vi "Process.vi"(0 "reference in":refnum<class "Simulated-PowerModule.lvclass">, 5 "error in":errorcluster) -> (14 "reference out":refnum<class "Simulated-PowerModule.lvclass">, 19 "error out":errorcluster)   [LabVIEW 2023, in "Simulated-PowerModule.lvlib" / "Simulated-PowerModule.lvclass"]
uses:
  Simulated-PowerModule.lvclass
  builds/PowerModuleInterface/PowerModuleInterface.lvlibp/Classes/PowerModule_interface/Slew Rates.ctl
  <instrlib>/HPS-17000/Client Facing Datatypes/Multi-Cycler Events.ctl
  <instrlib>/HPS-17000/Client Facing Datatypes/Heartbeat Event Data.ctl
  <instrlib>/HPS-17000/Client Facing Datatypes/Faults Event Data.ctl
  <instrlib>/HPS-17000/Client Facing Datatypes/Network Sync Event Data.ctl
  <instrlib>/HPS-17000/Client Facing Datatypes/Setpoint Stream Status Data.ctl
  builds/PowerModuleInterface/PowerModuleInterface.lvlibp/Classes/PowerModule_interface/Measurements.ctl
  <vilib>/addons/_JKI Toolkits/State Machine/_JKI_lib_State_Machine.llb/Conditional State String__jki_lib_state_machine.vi
  <vilib>/addons/_JKI Toolkits/State Machine/_JKI_lib_State_Machine.llb/Periodic Trigger__ogtk__JKI-SM__jki_lib_state_machine.vi
  Simulated-PowerModule.lvclass/Simulated-PowerModule.ctl
  <vilib>/Utility/SystemLogging/NI_SystemLogging.lvlib
  <instrlib>/HPS-17000/HPS-17000.lvclass
  builds/PowerModuleInterface/PowerModuleInterface.lvlibp/Classes/PowerModule_interface/PowerModuleInterface.lvclass
  <vilib>/measure/NI_MABase.lvlib
panel:
  in  "Main Tab Control":enum32{"CONFIG", "DEBUG"}(tab)
  out "Slew Rates":T1
  out "Last Command":string
  out "error info":errorcluster
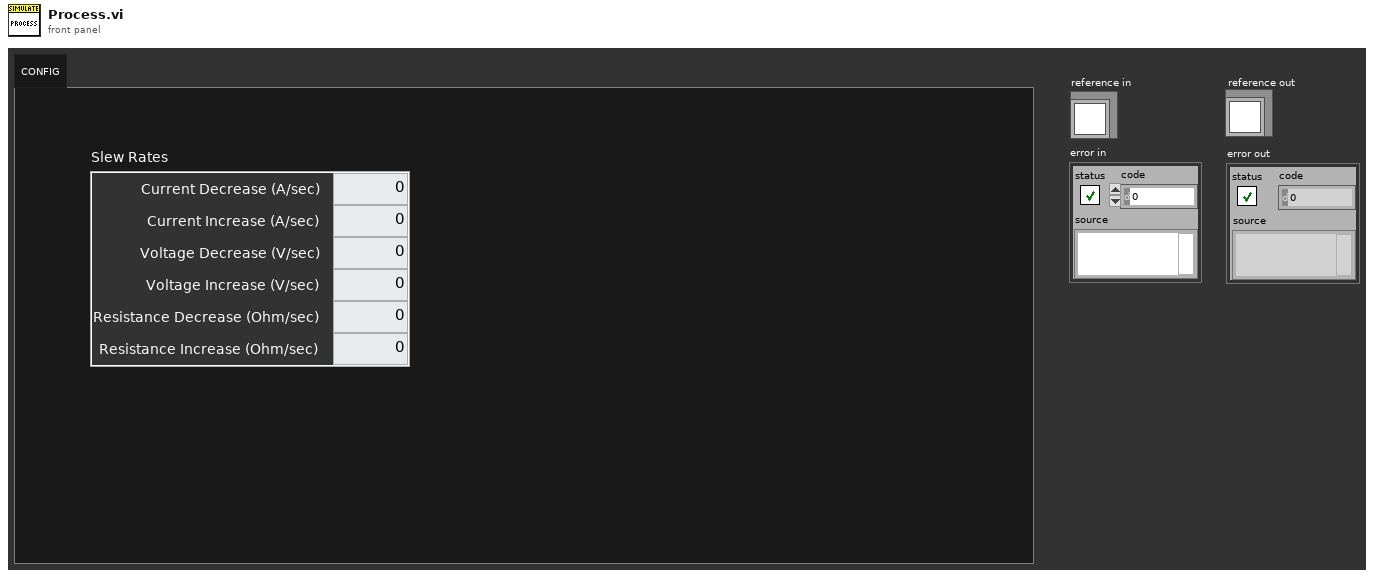
[diagram p1: front panel]
types:
  T1 = typedef "PowerModuleInterface.lvlibp/PowerModuleInterface.lvclass/Slew Rates.ctl" = cluster{"Current Decrease (A/sec)":dbl, "Current Increase (A/sec)":dbl, "Voltage Decrease (V/sec)":dbl, "Voltage Increase (V/sec)":dbl, "Resistance Decrease (Ohm/sec)":dbl, "Resistance Increase (Ohm/sec)":dbl}
  T2 = cluster{"Core":cluster{"Timeout":i32, "Events":cluster{"EventsToProcess":refnum<event-registration>, "UserEvents":refnum<event-registration>}, "EventFromProcess":refnum<user-event>, "ProcessSyncQueue":refnum<queue>, "QueueFromProcess":refnum<queue>, "Command":string, "Data":variant}}
  T3 = typedef "PowerModuleInterface.lvlibp/PowerModuleInterface.lvclass/Measurements.ctl" = cluster{"measured voltage (V)":dbl, "measured current (A)":dbl, "setpoint voltage (V)":dbl, "setpoint current (A)":dbl, "timestamp":dbl}
  T4 = enum32{"Invalid", "Standard", "Closed", "Hidden", "Minimized", "Maximized"}
  T5 = cluster{"EventsToProcess":refnum<event-registration>, "UserEvents":refnum<event-registration>}
  T6 = typedef "Simulated-PowerModule.lvlib/Simulated-PowerModule.lvclass/ObjectAttributes.ctl" = cluster{"JSON Config Path":path, "mode":T7, "Configuration":T8, "connected":bool, "reserved":bool, "energized":bool, "output enabled":bool, "setpoint":cluster{"voltage":dbl, "current":dbl, "resistance":dbl}, "last timestamp":i64, "measurement array":T3[], "profile":dbl[][], "step dt":i64, "measurement array size":u32}
  T7 = typedef "Simulated-PowerModule.lvlib/Simulated-PowerModule.lvclass/Mode.ctl" = u16
  T8 = typedef "Simulated-PowerModule.lvlib/Simulated-PowerModule.lvclass/Configuration.ctl" = cluster{"range":T9, "Limits":T10}
  T9 = typedef "PowerModuleInterface.lvlibp/PowerModuleInterface.lvclass/Range.ctl" = cluster{"Current Max (A)":dbl, "Current Min (A)":dbl, "Voltage Max (V)":dbl, "Voltage Min (V)":dbl}
  T10 = typedef "PowerModuleInterface.lvlibp/PowerModuleInterface.lvclass/Limits.ctl" = cluster{"Current Max (A)":dbl, "Current Min (A)":dbl, "Voltage Max (V)":dbl, "Voltage Min (V)":dbl, "Power Max (W)":dbl, "Power Min (W)":dbl}
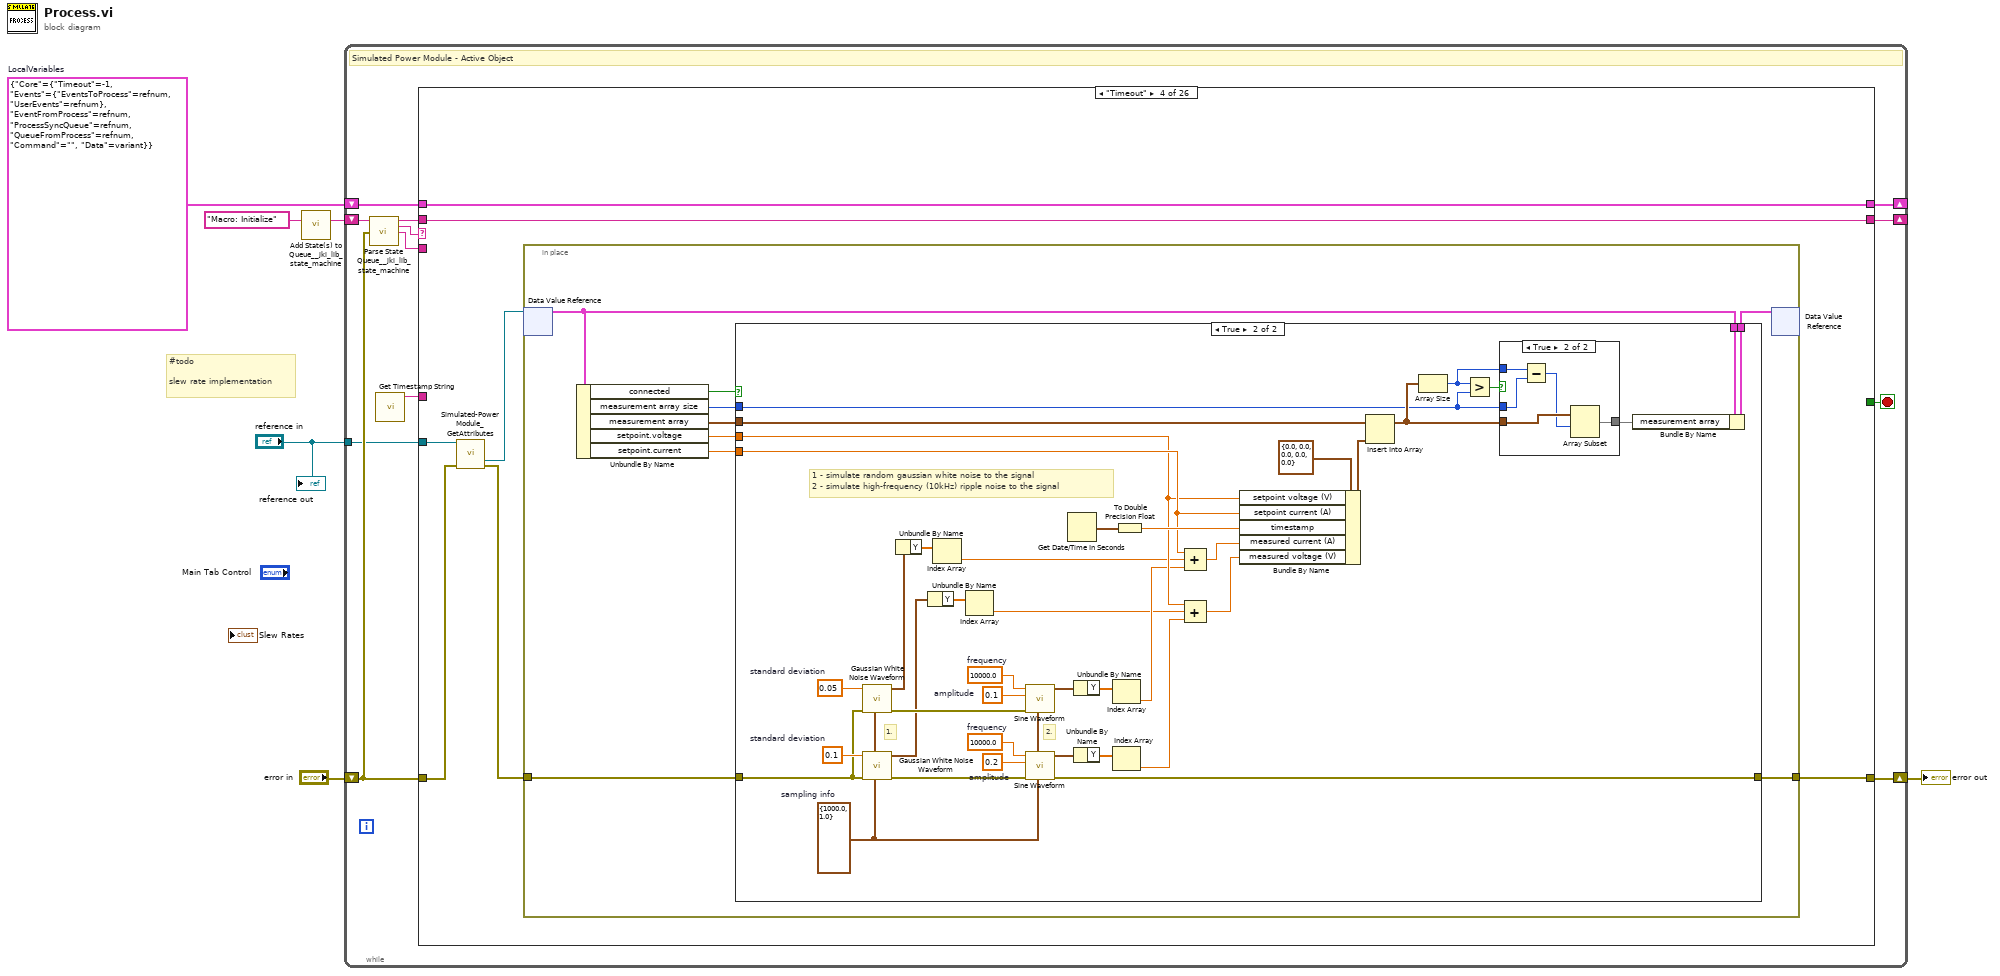
[diagram p0: block diagram]
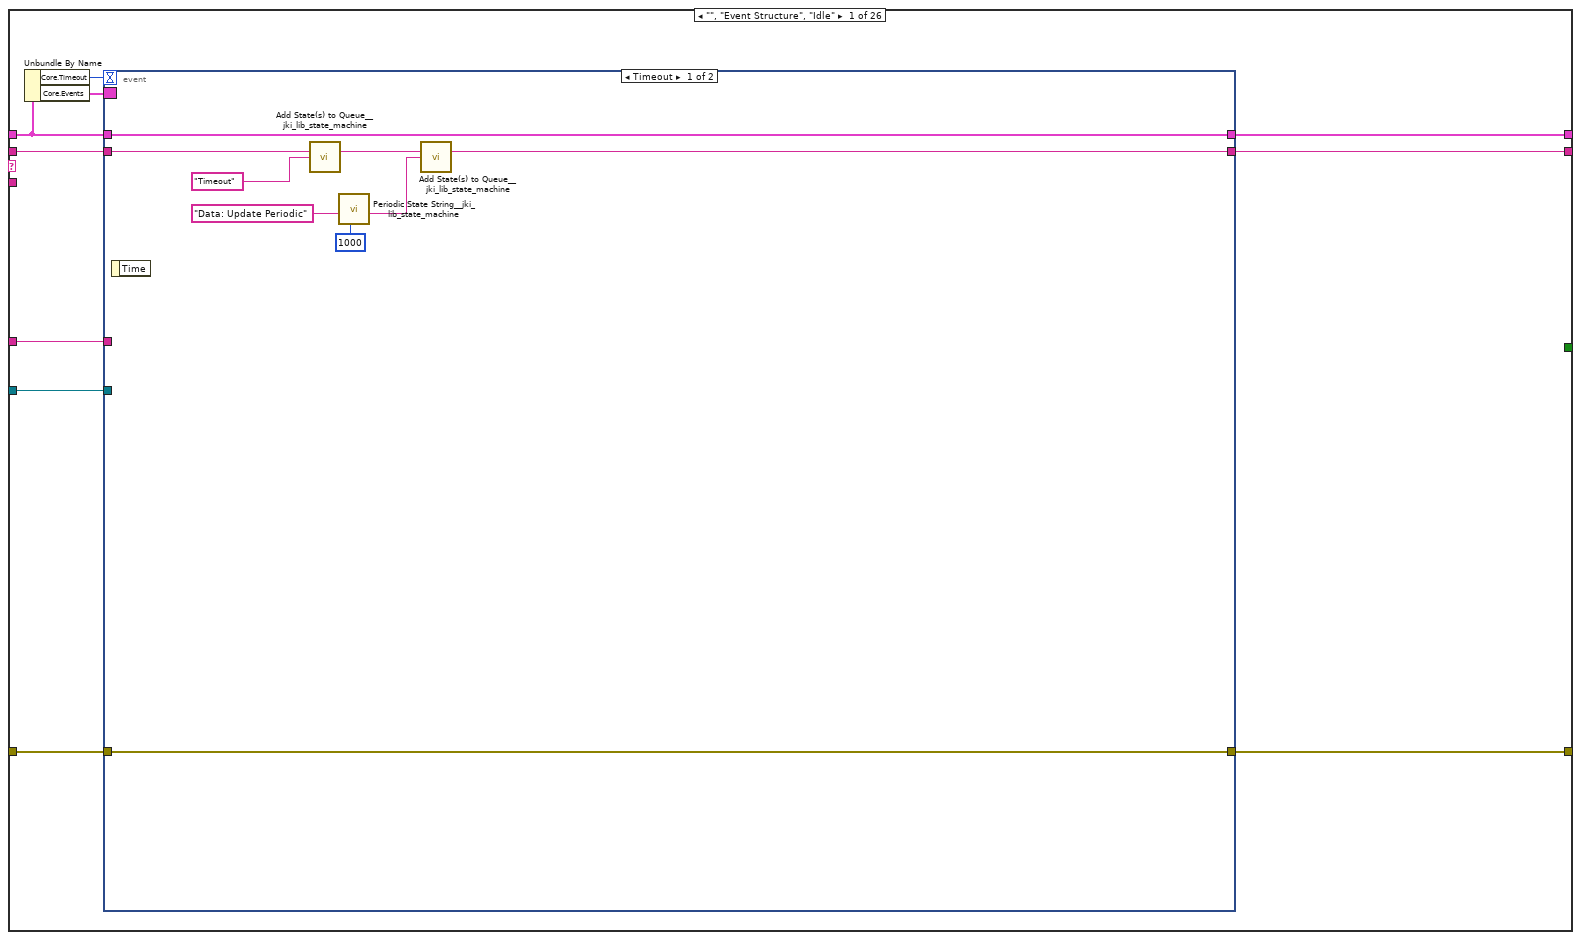
[diagram p2: hidden frame]
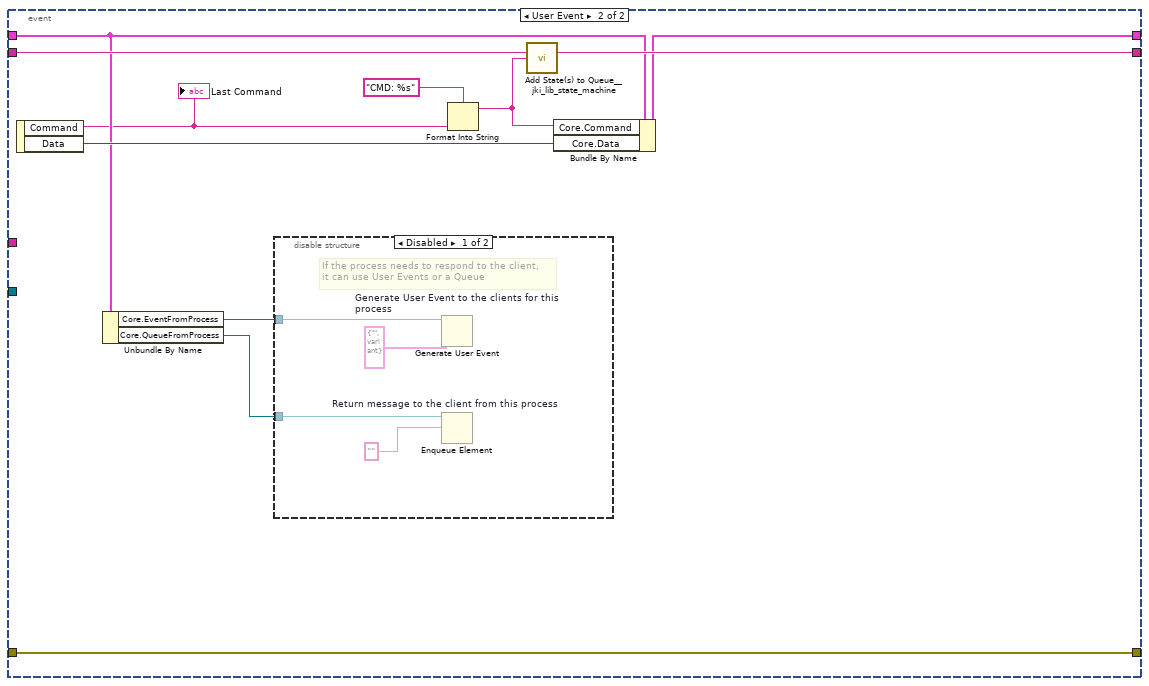
[diagram p3: hidden frame]
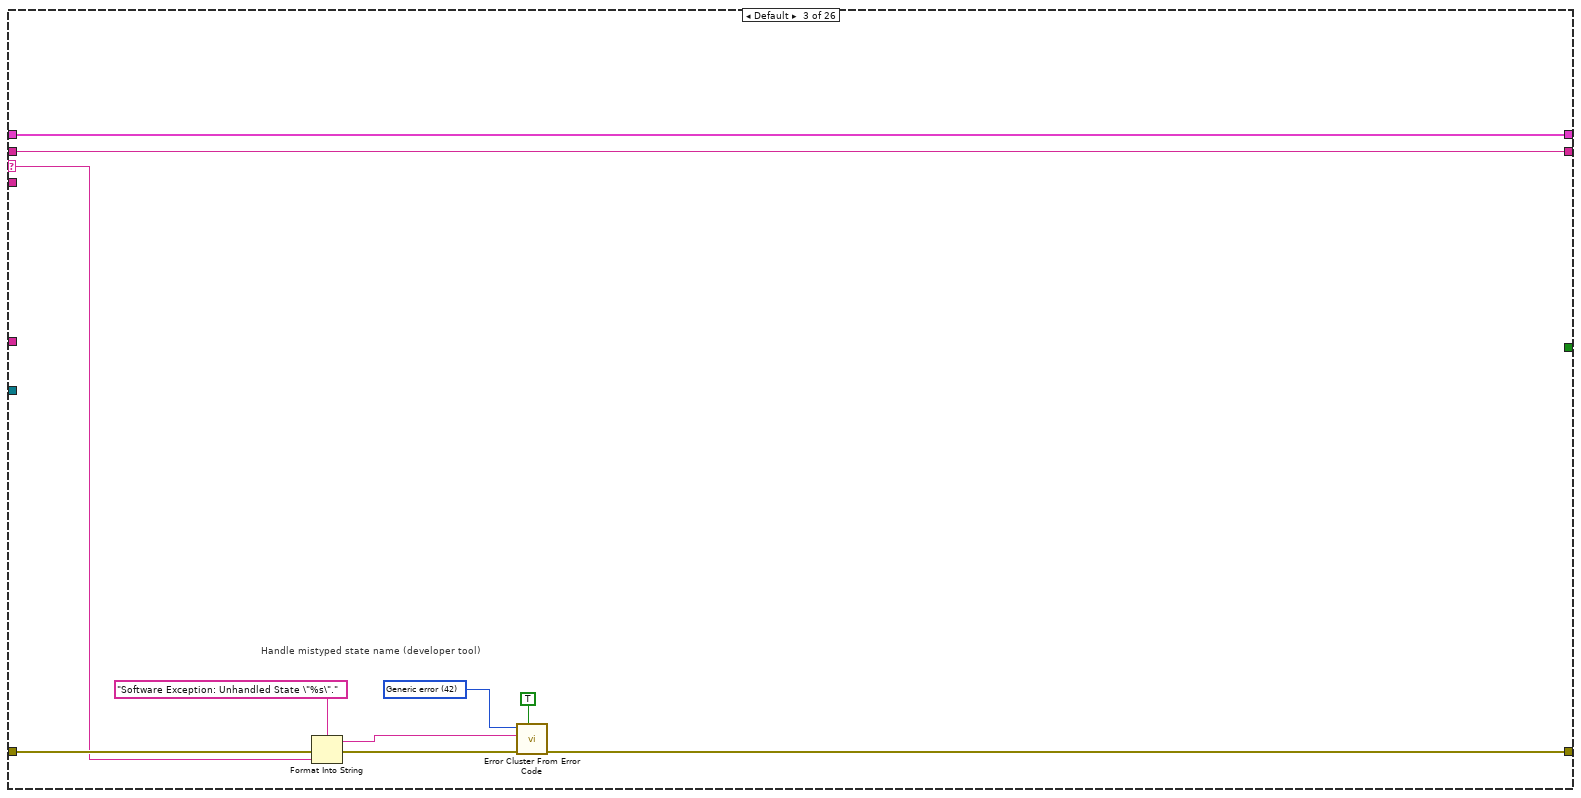
[diagram p6: hidden frame]
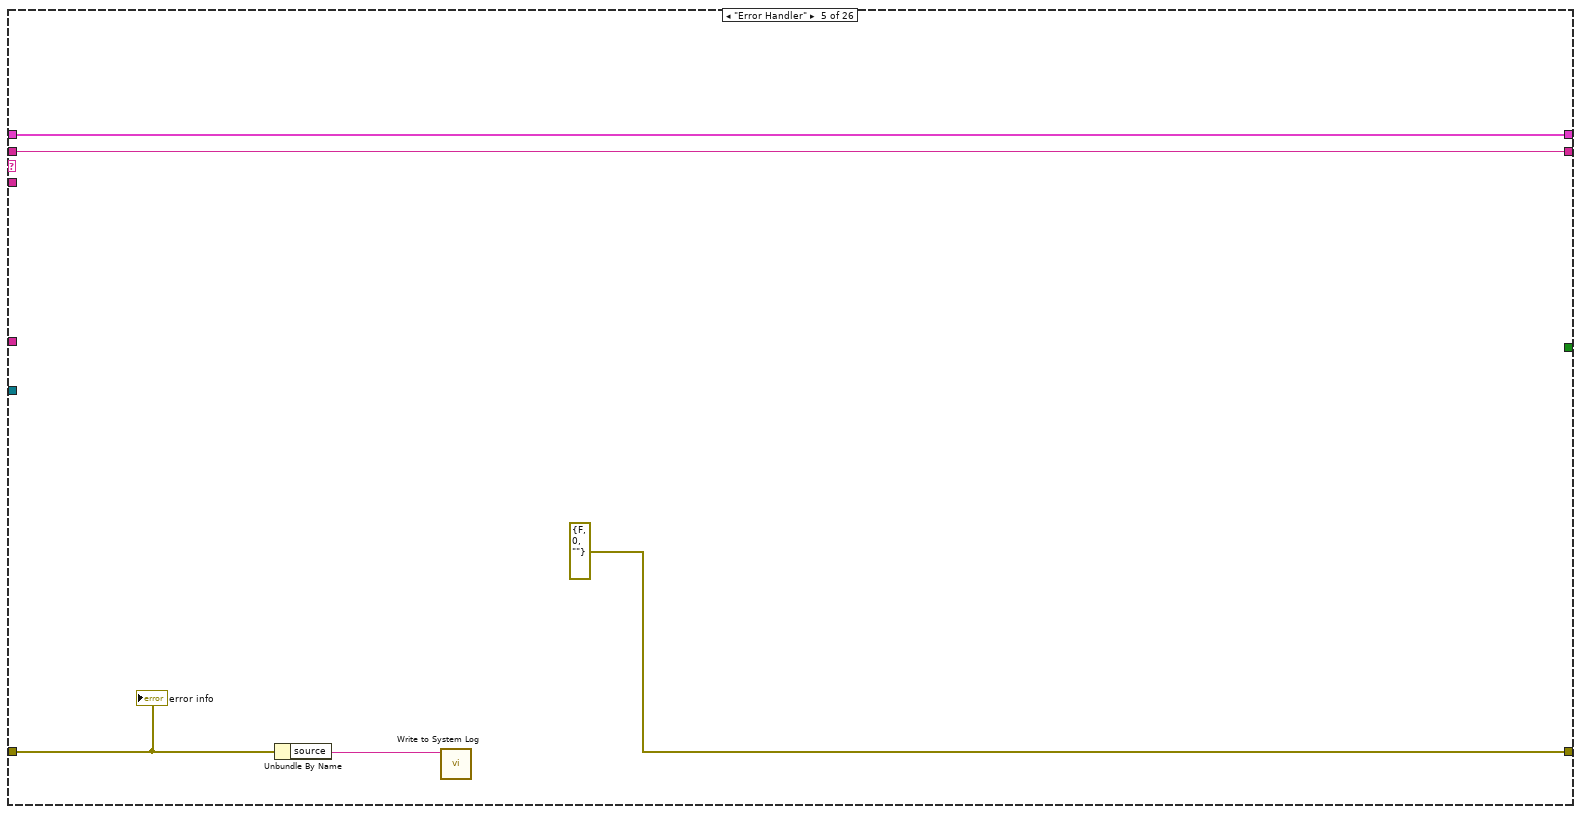
[diagram p9: hidden frame]
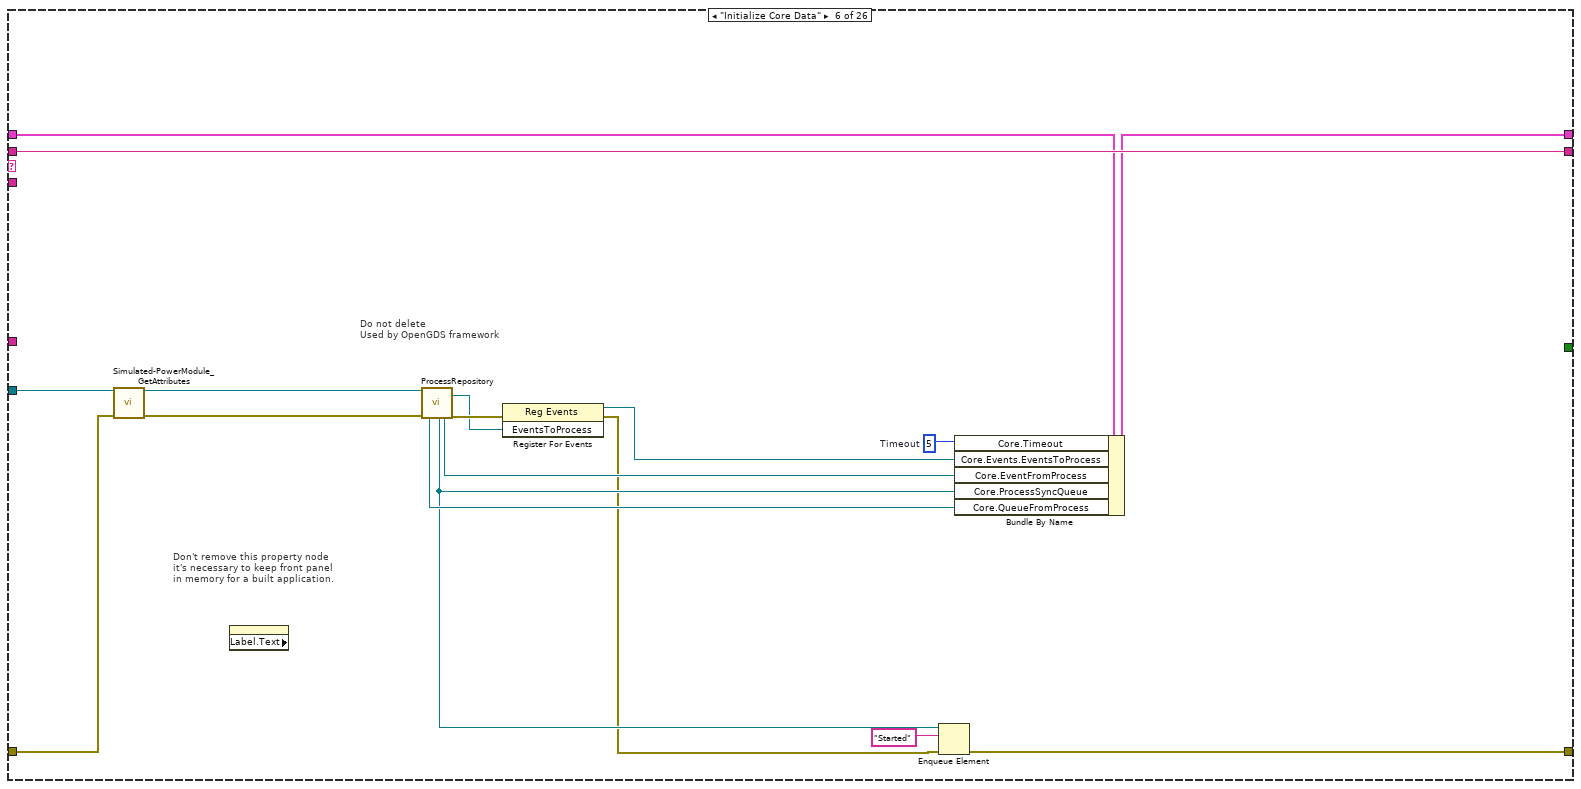
[diagram p10: hidden frame]
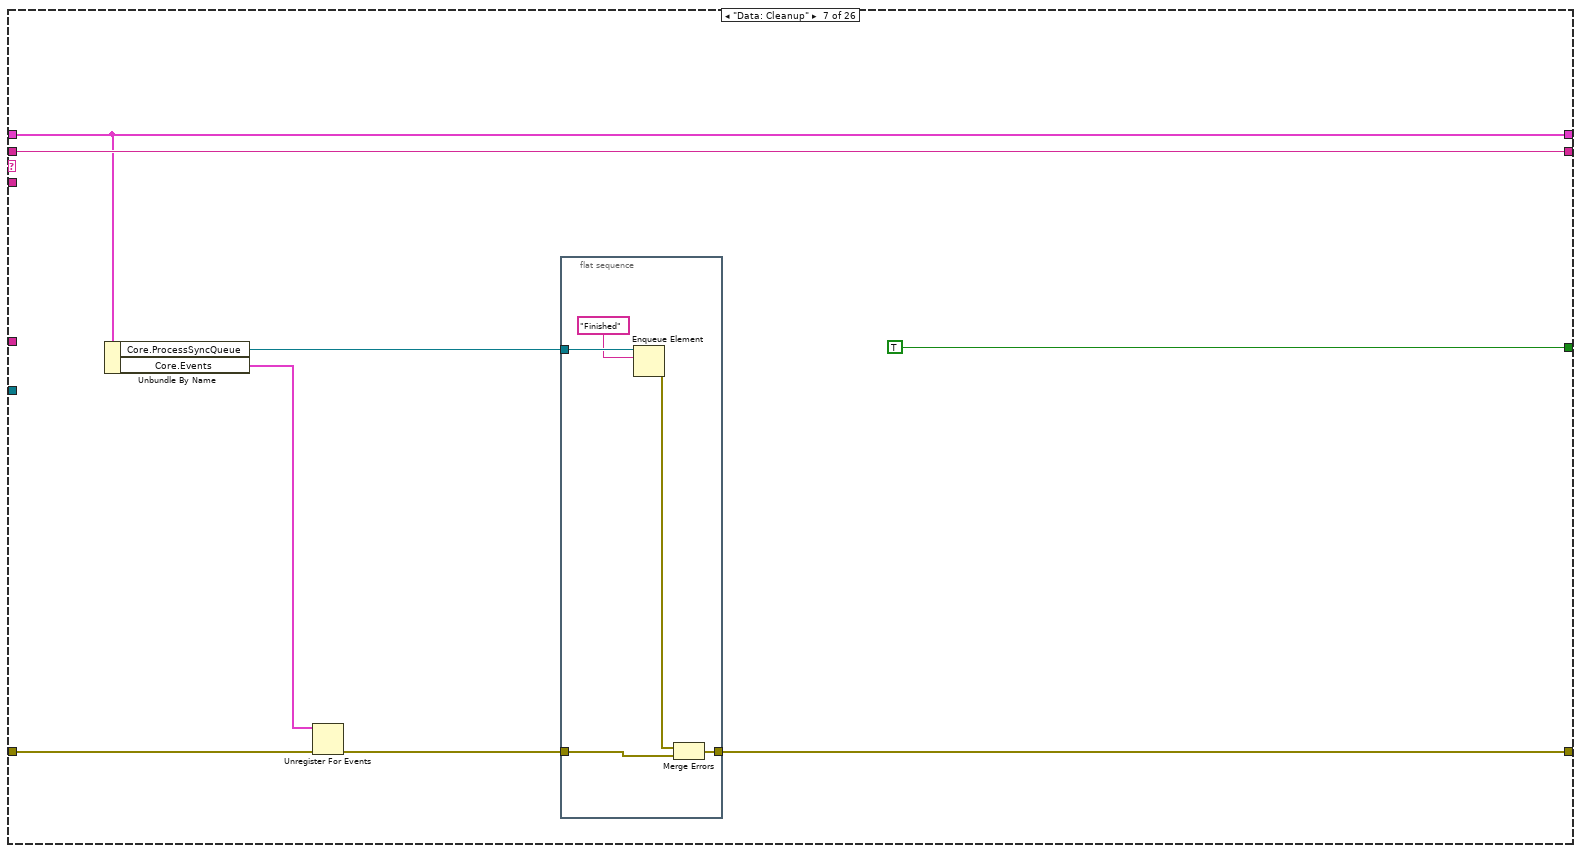
[diagram p11: hidden frame]
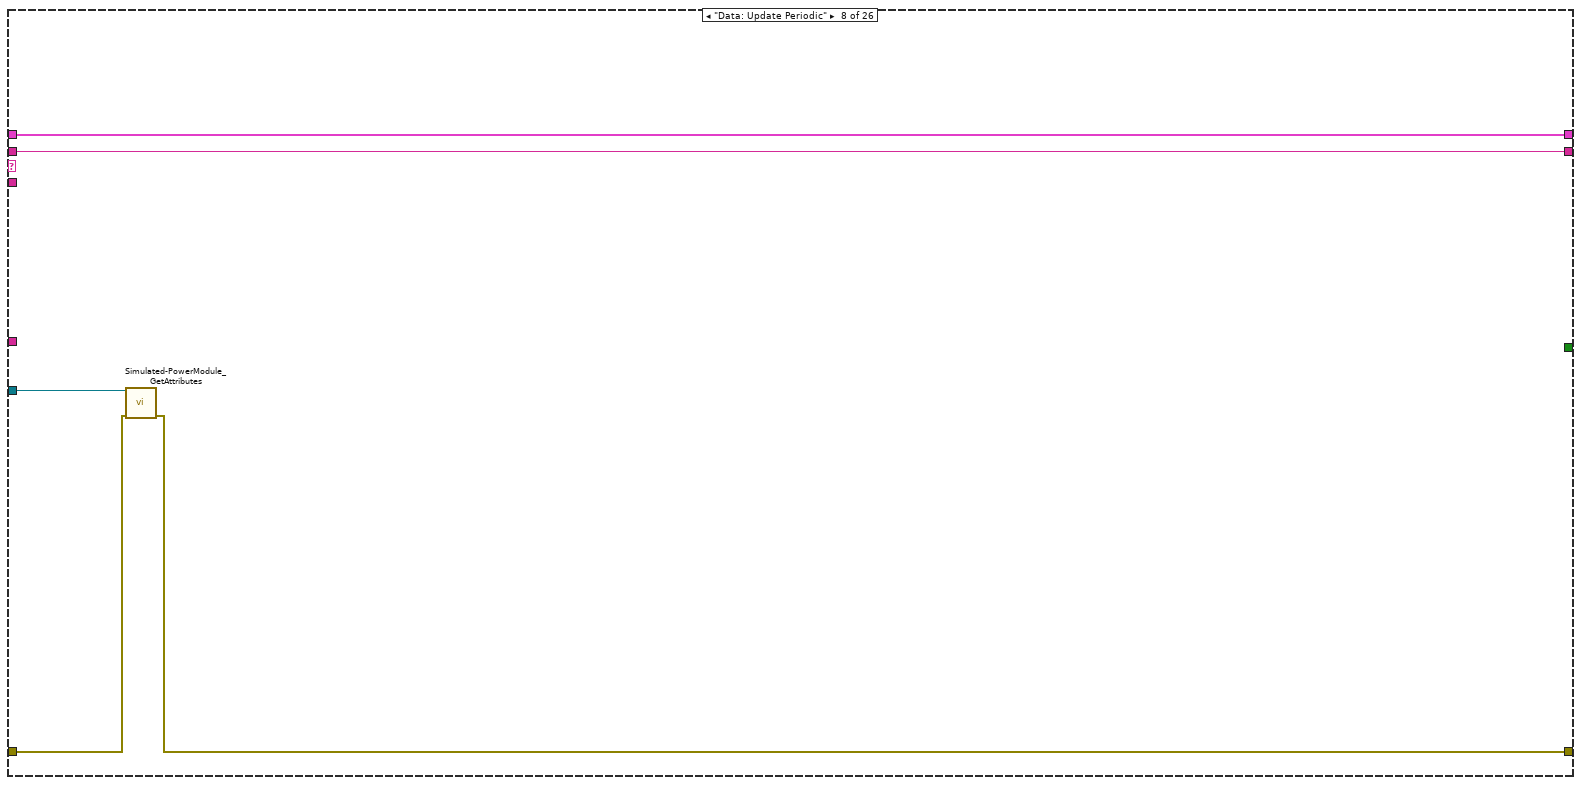
[diagram p12: hidden frame]
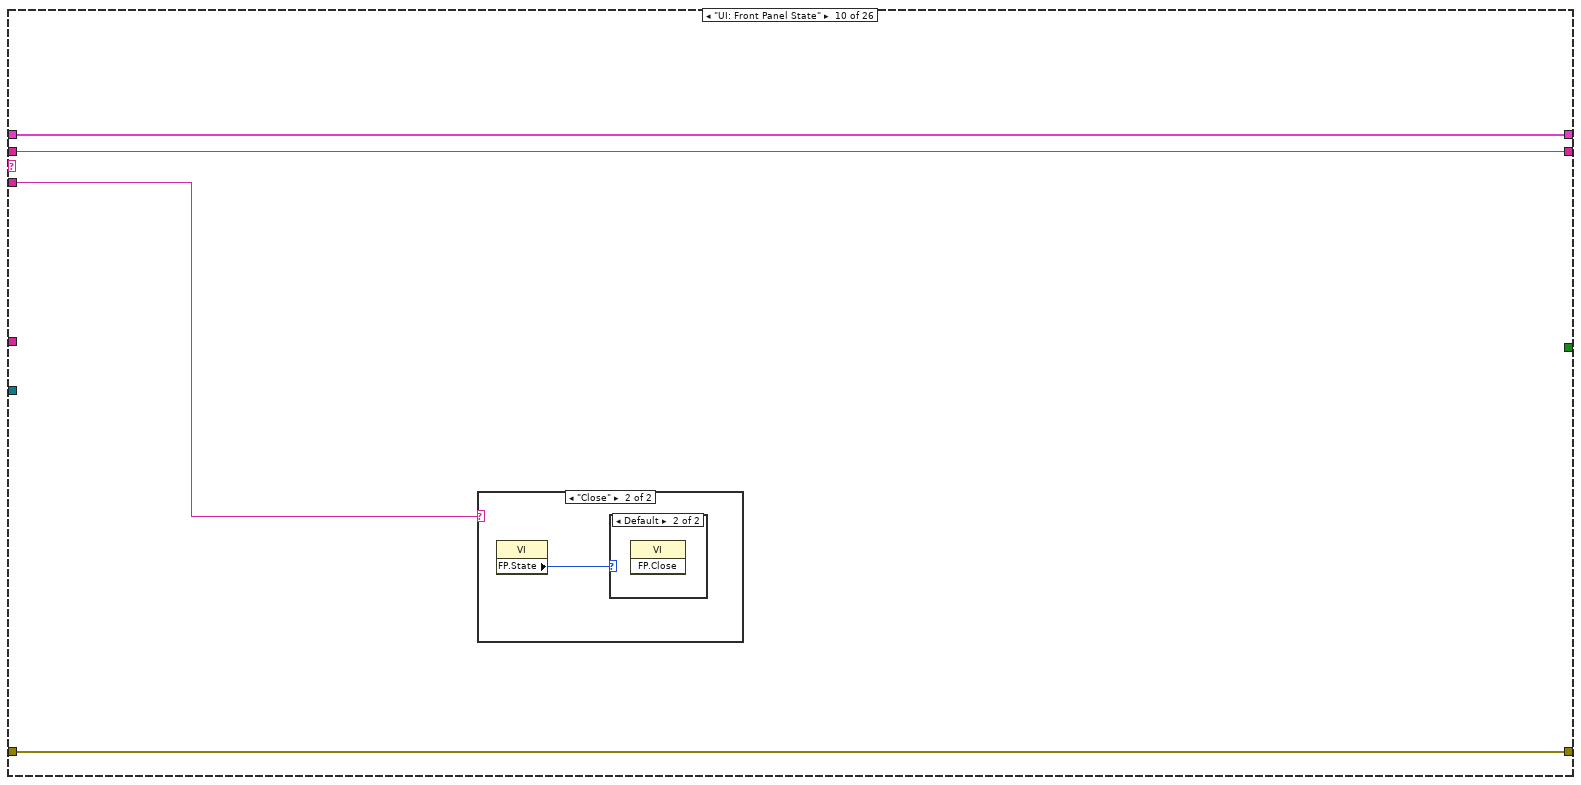
[diagram p14: hidden frame]
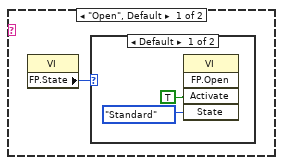
[diagram p15: hidden frame]
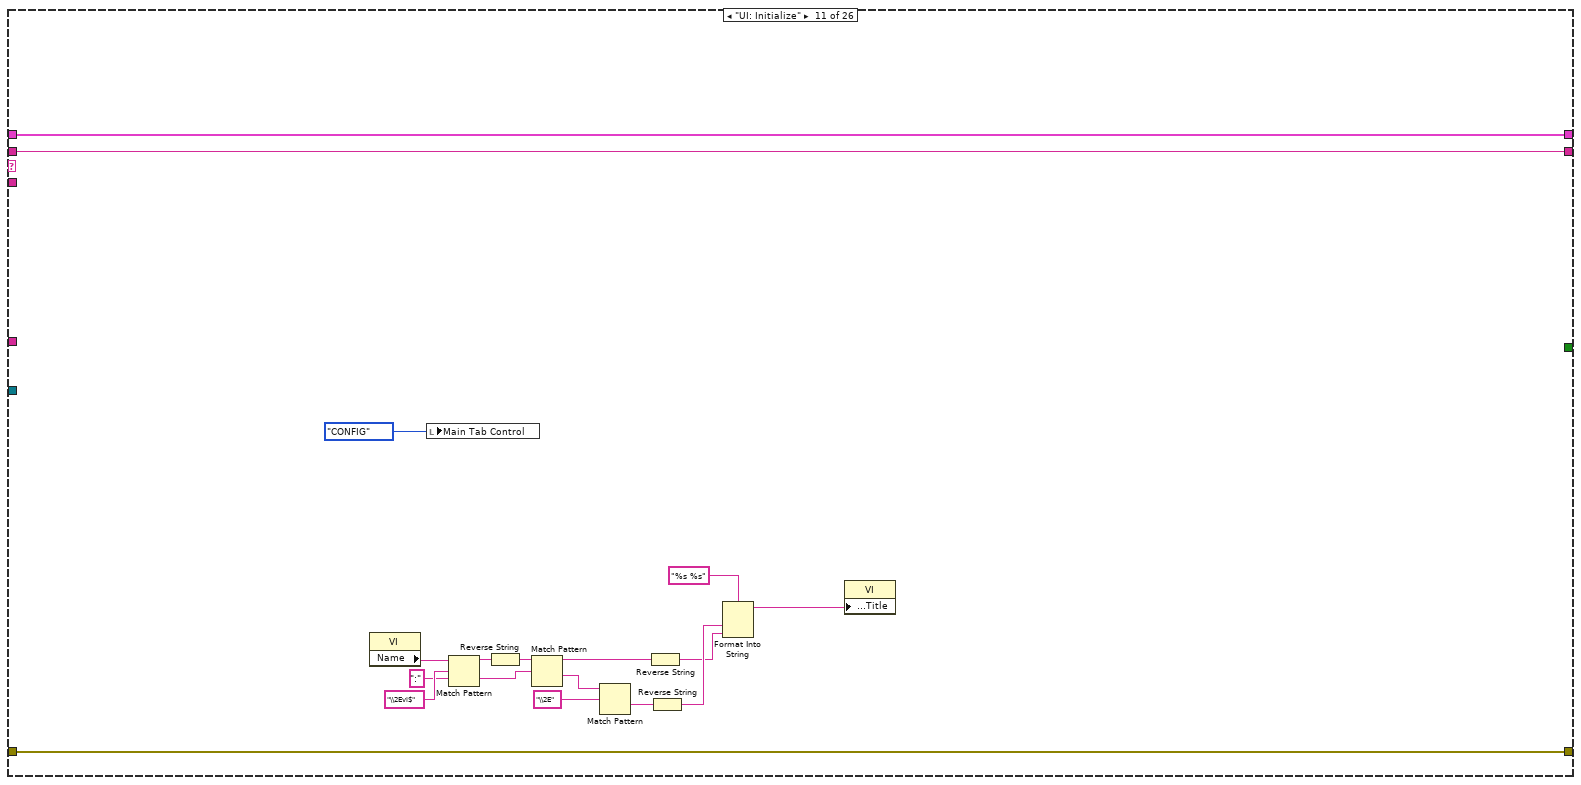
[diagram p18: hidden frame]
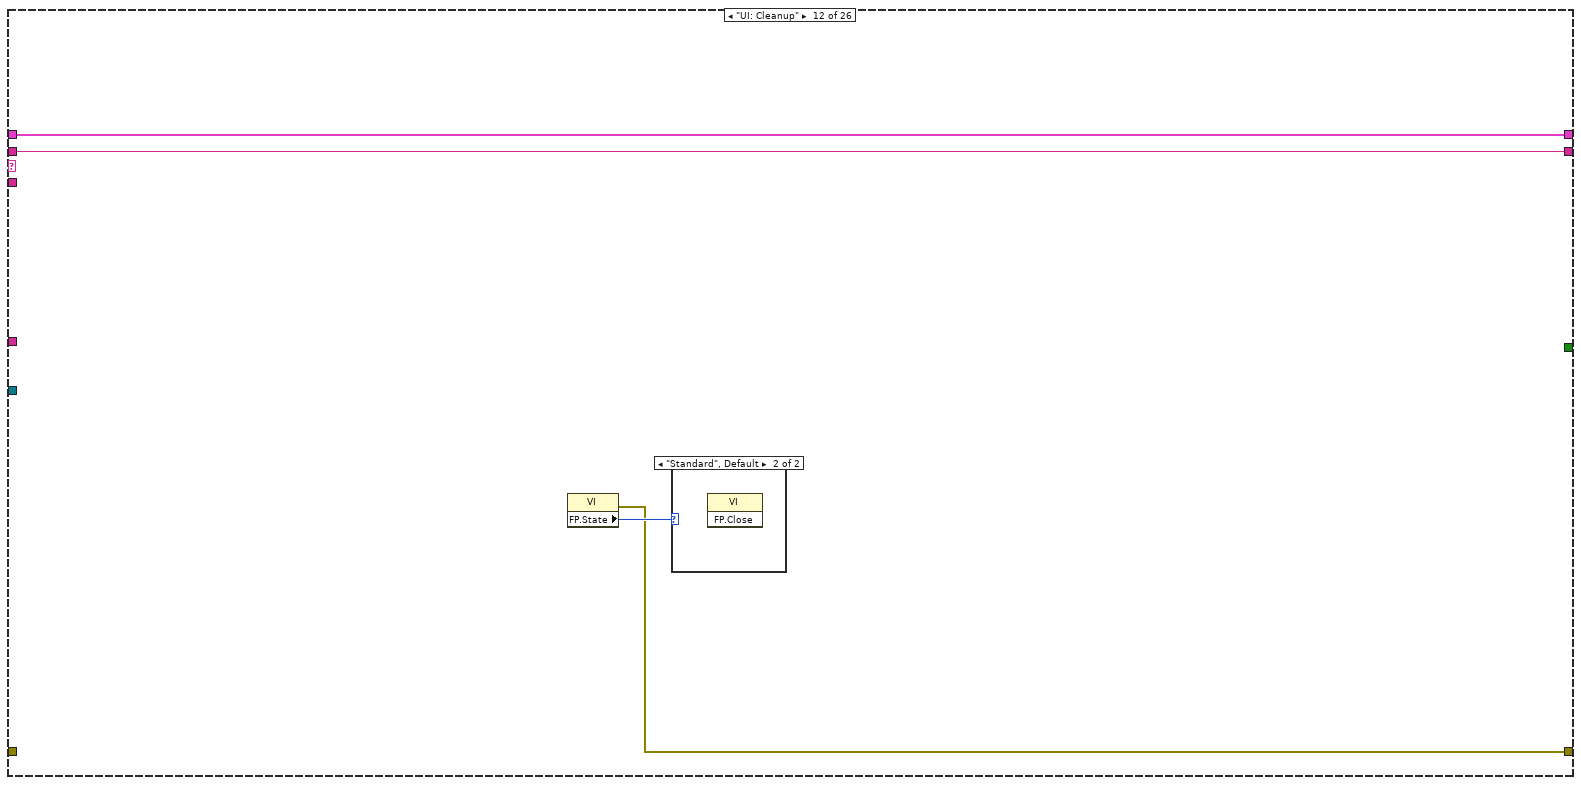
[diagram p19: hidden frame]
diagram:
  w6 = T2 {"Core"={"Timeout"=-1, "Events"={"EventsToProcess"=refnum, "UserEvents"=refnum}, "EventFromProcess"=refnum, "ProcessSyncQueue"=refnum, "QueueFromProcess"=refnum, "Command"="", "Data"=variant}}  # LocalVariables
  # "#todo\n\nslew rate implementation"
  n1 = call <vilib>:"Add State(s) to Queue__jki_lib_state_machine.vi"("State(s) in (\"\")"="Macro: Initialize" ("States Out")) -> ("States Out"=w2:string)  [unwired: 14 in]
  n2 = while {
    shift-right: [w17] -> w5
    shift-left: "error in" -> [w18]
    shift-right: [w10] -> _
    shift-left: w2 -> [w13]
    shift-right: [w16] -> _
    shift-left: w6 -> [w15]
    tunnel: "reference in" -> [w8]
    stop <- w9 stop-if-true
    # "Simulated Power Module - Active Object"
    n3 = call <vilib>:"Parse State Queue__jki_lib_state_machine.vi"("State Queue"=w13, "Error In (no error)"=w18) -> ("Remaining States"=w12:string, "Current State"=w14:string, "Arguments"=w11:string)  [unwired: 11 in]
    n4 = call "Get Timestamp String.vi"() -> ("date/time string"=w7:string)  [unwired: 11 in]
    n5 = case shown="\"Timeout\"" w14 {
      selector: w14 -> [_ _ w56 _ _ _ _ _ _ _ _ _ _ _ _ _ _ _ _ _ _ _ _ _ _ _]
      tunnel: w18 -> [w24 w55 w58 w69 w131 w135 w152 w165 w171 w172 w196 _ w202 w216 w219 w222 w227 w232 w235 w242 w251 w253 w263 w266 w271 w276]
      tunnel: [w22 w55 w57 w66 errorcluster {"status"=FALSE, "code"=0, "source"=""} ("error constant") w150 w154 w164 w171 w172 w196 w197 w201 w216 w219 w222 w227 w232 w235 w242 w246 w257 w263 w266 w271 w276] -> w17
      tunnel: [w28 w54 w65 w71 w133 w148 w155 w167 w170 w174 w188 w198 w205 w215 w218 w221 w226 w231 w234 w241 w250 w259 w262 w265 w270 w275] -> w16
      tunnel: w15 -> [w25 w54 w65 w71 w133 w147 w155 w167 w170 w174 w188 w198 w205 w215 w218 w221 w226 w231 w234 w241 w250 w259 w262 w265 w270 w275]
      tunnel: w12 -> [w27 w53 w64 w72 w132 w149 w158 w168 w169 w175 w195 w200 w204 w214 w217 w220 w225 w230 _ w240 w252 w260 w261 w264 w269 w274]
      tunnel: w11 -> [_ _ _ _ _ _ _ _ _ w173 _ _ w203 _ _ _ _ _ _ w237 _ _ _ _ _ _]
      tunnel: [w26 w53 w64 w72 w132 w149 w158 w168 w169 w175 w195 w200 w204 w214 w217 w220 w224 w229 "Macro: Exit" ("State(s) at Back (\"\")") w239 w252 w260 w261 w264 w267 w273] -> w10
      tunnel: [_ _ _ _ _ _ TRUE _ _ _ _ _ _ _ _ _ _ _ _ _ _ _ _ _ _ _] -> w9
      tunnel: w8 -> [w19 _ _ w70 _ w138 _ w166 _ _ _ _ _ _ _ _ _ _ _ _ _ _ _ _ _ _]
      tunnel: w7 -> [w20 _ _ _ _ _ _ _ _ _ _ _ _ _ _ _ _ _ _ _ _ _ _ _ _ _]
      frame "", "Event Structure", "Idle" {
        n6 = Unbundle By Name(w25) -> ("Core.Timeout"=w23:i32, "Core.Events"=w21:T5)
        n7 = event shown="[0] Timeout" {
          selector: w21 -> [_ _]
          dyn-events: _ -> [_ _]
          timeout: w23 -> [_ _]
          tunnel: w25 -> [w37 w41]
          tunnel: [w37 w46] -> w28
          tunnel: [w29 w48] -> w26
          tunnel: w27 -> [w36 w47]
          tunnel: [w34 w42] -> w22
          tunnel: w24 -> [w34 w42]
          tunnel: w20 -> [_ _]
          tunnel: w19 -> [_ _]
          event Timeout {
            n8 = event-data() -> ()  [unwired: 1 in, 1 out]
            n9 = call <vilib>:"Add State(s) to Queue__jki_lib_state_machine.vi"("State(s) in (\"\")"=w36, "State(s) at Back (\"\")"="Timeout" ("State(s) at Back (\"\")")) -> ("States Out"=w32:string)  [unwired: 13 in]
            n10 = call <vilib>:"Periodic State String__jki_lib_state_machine.vi"("Period (ms)"=u32 1000, "State"="Data: Update Periodic") -> ("State Out"=w31:string)  [unwired: 9 in]
            n11 = call <vilib>:"Add State(s) to Queue__jki_lib_state_machine.vi"("State(s) in (\"\")"=w32, "State(s) at Back (\"\")"=w31) -> ("States Out"=w29:string)  [unwired: 13 in]
          }
          event User Event {
            n12 = event-data() -> ("Command"=w39:string, "Data"=w45:variant)  [unwired: 1 in]
            "Last Command" <- w39
            n13 = Unbundle By Name(w41) -> ("Core.EventFromProcess"=w44:refnum<user-event>, "Core.QueueFromProcess"=w43:refnum<queue>)
            n14 = disable-structure shown="Disabled" {
              disable-tunnel: w44 -> [w52 _]
              disable-tunnel: w43 -> [w51 _]
              frame Disabled {
                # "If the process needs to respond to the client,\nit can use User Events or a Queue"
                n15 = Generate User Event "Generate User Event to the clients for this process"(user event=w52, event data cluster=cluster{"Command":string, "Data":variant} {"Command"="", "Data"=variant} ("event data")) -> ()  [unwired: 2 in, 2 out]
                n16 = Enqueue Element "Return message to the client from this process"(queue=w51, element="") -> ()  [unwired: 2 in, 3 out]
              }
              frame Enabled {
              }
            }
            n17 = Format Into String(format string="CMD: %s", w39) -> (resulting string=w38:string)  [unwired: 2 in, 1 out]
            n18 = call <vilib>:"Add State(s) to Queue__jki_lib_state_machine.vi"("State(s) in (\"\")"=w47, "State(s) at Back (\"\")"=w38) -> ("States Out"=w48:string)  [unwired: 13 in]
            n19 = Bundle By Name(cluster=w41, "Core.Command"=w38, "Core.Data"=w45) -> (w46:T2)
          }
        }
      }
      frame "---------- Core ----------" {
      }
      frame Default {
        w62 = 42 items=["No error", "Argument error", "Memory is full", "Out of zone", "End of file", "File already open", "Generic file I/O error", "File not found", "File permission error", "Disk is full", "Duplicate path", "Too many files open", "System feature not enabled", "Resource file not found", "Cannot add resource", "Resource not found", "Image not found", "Image memory error", "Pen does not exist", "Config type invalid", "Config token not found", "Config parse error", "Config memory error", "Bad external code format", "Bad external code offset", "External code not present", "Null window", "Destroy window error", "Null menu", "Print aborted", "Bad print record", "Print driver error", "Windows error during printing", "Memory error during printing", "Print dialog error", "Generic print error", "Invalid device refnum", "Device not found", "Device parameter error", "Device unit error", "Cannot open device", "Device call aborted", "Generic error", "Cancelled by user", "Object ID too low", "Object ID too high", "Object not in heap", "Unknown heap", "Unknown object (invalid DefProc)", "Unknown object (DefProc not in table)", "Message out of range", "Invalid (null) method", "Unknown message", "Manager call not supported", "Bad address", "Network operation in progress", "Network operation timed out", "Connection is busy", "Network attribute not supported", "Network error", "Address in use", "System out of memory", "Connection aborted", "Connection refused", "Not connected", "Already connected", "Connection closed", "Initialization error (interapplication manager)", "Bad occurrence", "Wait on unbound occurrence handler", "Occurrence queue overflow", "Datalog type conflict", "Unused", "Unrecognized type (interapplication manager)", "Memory corrupt", "Failed to make temporary DLL", "Old CIN version", "Drag socket not found", "Failed to load drop-object", "Failed to register OLE object", "Failed to release OLE object", "Format specifier type mismatch", "Unknown format specifier", "Too few format specifiers", "Too many format specifiers", "Scan failed", "Newer CIN version", "Error converting to variant", "Runtime menu error", "Password tampered", "Variant attribute not found", "Incompatible variant data type", "Event data is not available", "Event Store is not present", "Occurrence is not found", "Event Queue is not created", "Event info is not available", "Refnum passed is NULL", "Error retrieving Class GUID", "Error retrieving CoClass GUID", "Error retrieving TypeLib GUID.", "Bad built application magic bytes.", "Specific driver is different from the specific driver associated with the Logical Name.", "There is no session opened to the class driver.", "Max Error", "MAX - Error with config objects", "MAX - Error loading configuration", "MAX - Group not supported"]
        # "Handle mistyped state name (developer tool)"
        n20 = Format Into String(format string="Software Exception: Unhandled State \"%s\"." ("message"), error in=w58, w56) -> (resulting string=w61:string, error out=w60:errorcluster)  [unwired: 1 in]
        n21 = call <vilib>:"Error Cluster From Error Code.vi"("show call chain? (False)"=TRUE, "error in (no error)"=w60, "error message (\"\")"=w61, "error code (0)"=w62) -> ("error out"=w57:errorcluster)  [unwired: 5 in]
      }
      frame "Timeout" {
        # "High-Speed Measurement Stream"
        n22 = call "Simulated-PowerModule_GetAttributes.vi"("reference in"=w70, "Error In"=w69) -> ("DataRef"=w68:refnum<data-value>, "Error Out"=w67:errorcluster)  [unwired: 10 in, 2 out]
        n23 = in-place {
          in-place-border: w67 -> [w74]
          in-place-border: [w73] -> w66
          n24 = in-place-dvr #1(w68) -> (w80:T6)  [unwired: 1 out]
          n25 = Unbundle By Name(w80) -> ("connected"=w75:bool, "measurement array size"=w78:u32, "measurement array"=w79:T3[], "setpoint.voltage"=w76:dbl, "setpoint.current"=w77:dbl)
          n26 = case shown="True" w75 {
            tunnel: [w83 w122] -> w81
            tunnel: w80 -> [w83 w121]
            tunnel: w79 -> [_ w120]
            tunnel: w78 -> [_ w113]
            tunnel: w77 -> [_ w108]
            tunnel: w76 -> [_ w103]
            tunnel: w74 -> [w82 w96]
            tunnel: [w82 w106] -> w73
            frame False {
            }
            frame True {
              w95 = 0.05  # standard deviation
              w98 = 10000.0  # frequency
              w97 = 0.1  # amplitude
              w104 = 10000.0  # frequency
              w105 = 0.2  # amplitude
              w110 = 0.1  # standard deviation
              w93 = cluster{"Fs":dbl, "#s":dbl} {"Fs"=1000.0, "#s"=1.0}  # sampling info
              # "1 - simulate random gaussian white noise to the signal\n2 - simulate high-frequency (10kHz) ripple noise to the signal"
              # "2."
              # "1."
              n27 = call <vilib>:"Gaussian White Noise Waveform.vi"("sampling info"=w93, "error in (no error)"=w96, "standard deviation"=w95) -> ("error out"=w94:errorcluster, "signal out"=w89:waveform(dbl))  [unwired: 7 in]
              n28 = call <vilib>:"Gaussian White Noise Waveform.vi"("sampling info"=w93, "error in (no error)"=w96, "standard deviation"=w110) -> ("error out"=w107:errorcluster, "signal out"=w87:waveform(dbl))  [unwired: 7 in]
              n29 = Unbundle By Name(w89) -> ("Y"=w109:dbl[])
              n30 = Unbundle By Name(w87) -> ("Y"=w86:dbl[])
              n31 = Index Array(array=w109) -> (element=w92:dbl)  [unwired: 1 in]
              n32 = Index Array(array=w86) -> (element=w85:dbl)  [unwired: 1 in]
              n33 = call <vilib>:"Sine Waveform.vi"("sampling info"=w93, "error in (no error)"=w94, "amplitude"=w97, "frequency"=w98) -> ("signal out"=w90:waveform(dbl))  [unwired: 6 in, 1 out]
              n34 = call <vilib>:"Sine Waveform.vi"("sampling info"=w93, "error in (no error)"=w107, "amplitude"=w105, "frequency"=w104) -> ("error out"=w106:errorcluster, "signal out"=w100:waveform(dbl))  [unwired: 6 in]
              n35 = Get Date/Time In Seconds() -> (seconds since 1Jan1904=w112:timestamp)
              n36 = Unbundle By Name(w90) -> ("Y"=w91:dbl[])
              n37 = Unbundle By Name(w100) -> ("Y"=w99:dbl[])
              n38 = Index Array(array=w91) -> (element=w88:dbl)  [unwired: 1 in]
              n39 = Index Array(array=w99) -> (element=w84:dbl)  [unwired: 1 in]
              n40 = To Double Precision Float(number=w112) -> (double precision float=w111:dbl)
              n41 = Compound Arithmetic op=ADD(w108, w92, w88) -> (w102:dbl)
              n42 = Compound Arithmetic op=ADD(w103, w85, w84) -> (w101:dbl)
              n43 = Bundle By Name(cluster=T3 {"measured voltage (V)"=0.0, "measured current (A)"=0.0, "setpoint voltage (V)"=0.0, "setpoint current (A)"=0.0, "timestamp"=0.0} ("Measurements"), "setpoint voltage (V)"=w103, "setpoint current (A)"=w108, "timestamp"=w111, "measured current (A)"=w102, "measured voltage (V)"=w101) -> (w115:T3)
              n44 = Insert Into Array(array=w120, new element=w115) -> (w117:T3[])  [unwired: 1 in]
              n45 = Array Size(array=w117) -> (size(s)=w114:i32)
              n46 = Greater?(x=w114, y=w113) -> (0:w116:bool)
              n47 = case shown="True" w116 {
                tunnel: [w123 w128] -> w119
                tunnel: w117 -> [w123 w127]
                tunnel: w114 -> [_ w126]
                tunnel: w113 -> [_ w125]
                frame False {
                }
                frame True {
                  n48 = Subtract(x=w126, y=w125) -> (x-y=w124:u32)
                  n49 = Array Subset(array=w127, index=w124) -> (w128:T3[])  [unwired: 1 in]
                }
              }
              n50 = Bundle By Name(cluster=w121, "measurement array"=w119) -> (w122:T6)
            }
          }
          n51 = in-place-dvr #1(w81) -> ()  [unwired: 2 out]
        }
      }
      frame "Error Handler" {
        n52 = Unbundle By Name(w131) -> ("source"=w129:string)
        n53 = call <vilib>:"Write to System Log.vi"("message"=w129) -> ()  [unwired: 10 in, 1 out]
        "error info" <- w131
      }
      frame "Initialize Core Data" {
        w139 = 5  # Timeout
        # "Do not delete\nUsed by OpenGDS framework"
        # "Don't remove this property node\nit's necessary to keep front panel\nin memory for a built application."
        # "Template created by VI Technologies"
        n54 = call "Simulated-PowerModule_GetAttributes.vi"("reference in"=w138, "Error In"=w135) -> ("reference out"=w136:refnum<class "Simulated-PowerModule.lvclass">, "Error Out"=w137:errorcluster)  [unwired: 10 in, 2 out]
        n55 = property on="reference in" class="LVClassControl (strict)" props=["Label", "Text"]() -> ()  [unwired: 2 in, 3 out]
        n56 = call "ProcessRepository.vi"("reference in"=w136, "Error In"=w137) -> ("QueueFromProcess"=w142:refnum<queue>, "ProcessSyncQueue"=w140:refnum<queue>, "EventFromProcess"=w143:refnum<user-event>, "EventsToProcess"=w145:refnum<user-event>, "Error Out"=w146:errorcluster)  [unwired: 10 in, 3 out]
        n57 = register-events(error in=w146, w145) -> (reference out=w144:refnum<event-registration>, error out=w134:errorcluster)  [unwired: 1 in]
        n58 = Enqueue Element(queue=w140, element="Started", error in (no error)=w134) -> (error out=w150:errorcluster)  [unwired: 1 in, 2 out]
        n59 = Bundle By Name(cluster=w147, "Core.Timeout"=w139, "Core.Events.EventsToProcess"=w144, "Core.EventFromProcess"=w143, "Core.ProcessSyncQueue"=w140, "Core.QueueFromProcess"=w142) -> (w148:T2)
      }
      frame "Data: Cleanup" {
        n60 = Unbundle By Name(w155) -> ("Core.ProcessSyncQueue"=w156:refnum<queue>, "Core.Events"=w153:T5)
        n61 = Unregister For Events(event registration refnum=w153, error in=w152) -> (error out=w151:errorcluster)
        n62 = flat-sequence {
          tunnel: [w162] -> w154
          tunnel: w156 -> [w161]
          tunnel: w151 -> [w160]
          frame #0 {
            n63 = Enqueue Element(queue=w161, element="Finished") -> (error out=w163:errorcluster)  [unwired: 2 in, 2 out]
            n64 = Merge Errors(w163, w160) -> (w162:errorcluster)
          }
        }
      }
      frame "Data: Update Periodic" {
        n65 = call "Simulated-PowerModule_GetAttributes.vi"("reference in"=w166, "Error In"=w165) -> ("Error Out"=w164:errorcluster)  [unwired: 10 in, 3 out]
      }
      frame "---------- UI ----------" {
      }
      frame "UI: Front Panel State" {
        n66 = case shown="\"Close\"" w173 {
          frame "Open", Default {
            n67 = property class="VI"() -> ("FP.State"=w176:T4)  [unwired: 2 in, 2 out]
            n68 = case shown="Default" w176 {
              frame Default {
                n69 = invoke class="VI" method="FP.Open"("Activate"=TRUE, "State"=T4."Standard") -> ()  [unwired: 3 in, 5 out]
              }
              frame "Standard" {
              }
            }
          }
          frame "Close" {
            n70 = property class="VI"() -> ("FP.State"=w179:T4)  [unwired: 2 in, 2 out]
            n71 = case shown="Default" w179 {
              frame "Closed" {
              }
              frame Default {
                n72 = invoke class="VI" method="FP.Close"() -> ()  [unwired: 3 in, 3 out]
              }
            }
          }
        }
      }
      frame "UI: Initialize" {
        n73 = property class="VI"() -> ("Name"=w194:string)  [unwired: 2 in, 2 out]
        n74 = local write "Main Tab Control"(enum32{"CONFIG", "DEBUG"}."CONFIG" ("Main Tab Control")) -> ()
        n75 = Match Pattern(string=w194, regular expression="\\2Evi$") -> (before substring=w192:string)  [unwired: 1 in, 3 out]
        n76 = Reverse String(1:w192) -> (0:w191:string)
        n77 = Match Pattern(string=w191, regular expression=":") -> (before substring=w189:string, after substring=w187:string)  [unwired: 1 in, 2 out]
        n78 = Match Pattern(string=w187, regular expression="\\2E") -> (after substring=w185:string)  [unwired: 1 in, 3 out]
        n79 = Reverse String(1:w189) -> (0:w183:string)
        n80 = Reverse String(1:w185) -> (0:w184:string)
        n81 = Format Into String(format string="%s %s", w184, w183) -> (resulting string=w182:string)  [unwired: 2 in, 1 out]
        n82 = property class="VI"("Front Panel.Title"=w182) -> ()  [unwired: 2 in, 2 out]
      }
      frame "UI: Cleanup" {
        n83 = property class="VI"() -> (error out=w197:errorcluster, "FP.State"=w199:T4)  [unwired: 2 in, 1 out]
        n84 = case shown="\"Standard\", Default" w199 {
          frame "Closed" {
          }
          frame "Standard", Default {
            n85 = invoke class="VI" method="FP.Close"() -> ()  [unwired: 3 in, 3 out]
          }
        }
      }
      frame "UI: Cursor Set" {
        # "Argument"
        # "Set and Unset Cursor Busy.\n(Usage: \"UI: Cursor Set >> Busy|Idle\")"
        n86 = disable-structure shown="TARGET_TYPE==Windows, Default" {
          disable-tunnel: w203 -> [w208 _]
          disable-tunnel: w202 -> [w207 w213]
          disable-tunnel: [w206 w213] -> w201
          frame condition #0 (active) {
            n87 = case shown="\"Busy\"" w208 {
              tunnel: w207 -> [w210 w212]
              tunnel: [w209 w211] -> w206
              frame "Idle", Default {
                n88 = call <vilib>:"Unset Busy.vi"("error in (no error)"=w210) -> ("error out"=w209:errorcluster)  [unwired: 10 in]
              }
              frame "Busy" {
                n89 = call <vilib>:"Set Busy.vi"("error in (no error)"=w212) -> ("error out"=w211:errorcluster)  [unwired: 9 in, 1 out]
              }
            }
          }
          frame condition #1 {
          }
        }
      }
      frame "---------- CMD ----------" {
      }
      frame "CMD: Connect" {
      }
      frame "CMD: Disconnect" {
      }
      frame "CMD: Reserve" {
        # "Reserve Macro\n(This is called when we reserve the Simulated PMOD)"
        n90 = call <vilib>:"Add State(s) to Queue__jki_lib_state_machine.vi"("State(s) in Front (\"\")"="", "State(s) in (\"\")"=w225) -> ("States Out"=w224:string)  [unwired: 13 in]
      }
      frame "CMD: Unreserve" {
        # "Unreserve Macro\n(This is called when we unreserve the Simulated PMOD)"
        n91 = call <vilib>:"Add State(s) to Queue__jki_lib_state_machine.vi"("State(s) in Front (\"\")"="", "State(s) in (\"\")"=w230) -> ("States Out"=w229:string)  [unwired: 13 in]
      }
      frame "CMD: Exit" {
      }
      frame "CMD: Front Panel State" {
        n92 = Format Into String(format string="UI: Front Panel State>>%s" ("string"), w237) -> (resulting string=w236:string)  [unwired: 2 in, 1 out]
        n93 = call <vilib>:"Add State(s) to Queue__jki_lib_state_machine.vi"("State(s) in (\"\")"=w240, "State(s) at Back (\"\")"=w236) -> ("States Out"=w239:string)  [unwired: 13 in]
      }
      frame "CMD: Write Slew Rates" {
        n94 = Unbundle By Name(w250) -> ("Core.QueueFromProcess"=w247:refnum<queue>, "Core.Data"=w249:variant)
        n95 = Variant To Data(error in=w251, type=T1 {"Current Decrease (A/sec)"=0.0, "Current Increase (A/sec)"=0.0, "Voltage Decrease (V/sec)"=0.0, "Voltage Increase (V/sec)"=0.0, "Resistance Decrease (Ohm/sec)"=0.0, "Resistance Increase (Ohm/sec)"=0.0} ("Slew Rates"), Variant=w249) -> (data=w245:T1, error out=w244:errorcluster)
        n96 = local write "Slew Rates"(w245) -> ()
        n97 = Enqueue Element(queue=w247, element="", error in (no error)=w244) -> (error out=w246:errorcluster)  [unwired: 1 in, 2 out]
      }
      frame "CMD: Read Slew Rates" {
        n98 = Unbundle By Name(w259) -> ("Core.QueueFromProcess"=w258:refnum<queue>)
        n99 = local read "Slew Rates"() -> (w254:T1)
        n100 = Flatten To String(anything=w254, error in (no error)=w253) -> (data string=w255:string, error out=w256:errorcluster)  [unwired: 2 in, 1 out]
        n101 = Enqueue Element(queue=w258, element=w255, error in (no error)=w256) -> (error out=w257:errorcluster)  [unwired: 1 in, 2 out]
      }
      frame "CMD: Acknowledge" {
      }
      frame "---------- Macro ----------" {
      }
      frame "Macro: Initialize" {
        n102 = call <vilib>:"Add State(s) to Queue__jki_lib_state_machine.vi"("State(s) in Front (\"\")"="Initialize Core Data\nUI: Initialize" ("States Out"), "State(s) in (\"\")"=w269) -> ("States Out"=w267:string)  [unwired: 13 in]
      }
      frame "Macro: Exit" {
        # "Exit Macro\n(This is called once, when the VI exits)"
        n103 = call <vilib>:"Add State(s) to Queue__jki_lib_state_machine.vi"("State(s) in Front (\"\")"="UI: Cleanup\nData: Cleanup" ("State(s) at Back (\"\")"), "State(s) in (\"\")"=w274) -> ("States Out"=w273:string)  [unwired: 13 in]
      }
    }
  }
  "error out" <- w5
  "reference out" <- "reference in"
